vi "PWM.vi"(8 "Detener el PWM":bool, 9 "milliseconds to wait":u32, 10 "Ciclo de Trabajo":dbl(knob) scale=0.0..100.0, 11 "Frecuencia":dbl(knob) scale=0.0..100.0) -> (3 "Señal PWM":dbl(graph))   [LabVIEW 2018]
panel:
  # "Señal PWM"
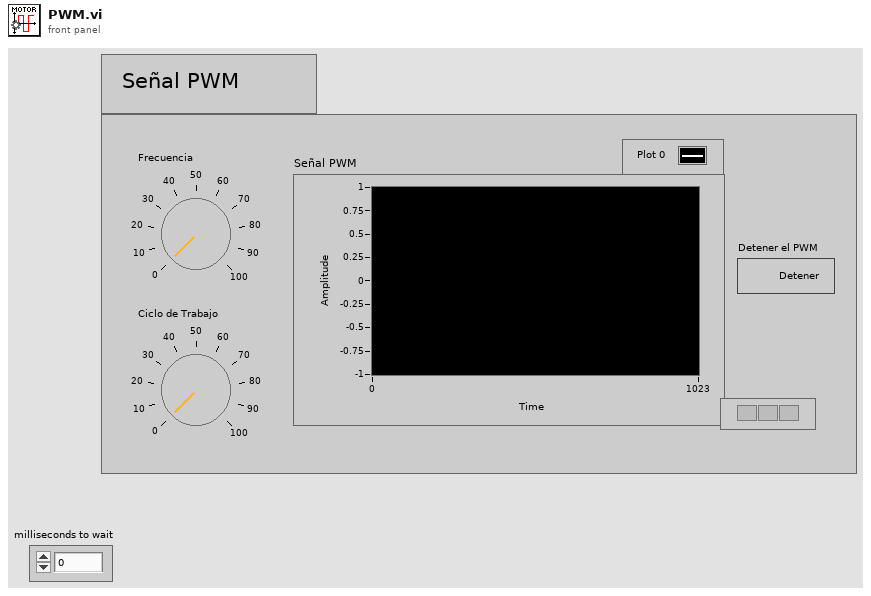
[diagram p1: front panel]
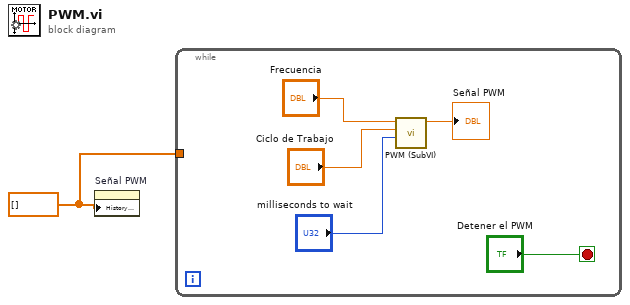
[diagram p0: block diagram]
diagram:
  w1 = dbl[] [] ("History Data")
  n1 = property on="Señal PWM" class="WFChart (strict)"("History Data"=w1) -> ()  [unwired: 2 in, 2 out]
  n2 = while {
    tunnel: w1 -> [_]
    stop <- "Detener el PWM" stop-if-true
    n3 = call "PWM (SubVI).vi"("milliseconds to wait"="milliseconds to wait", "Ciclo de Trabajo"="Ciclo de Trabajo", "Frecuencia"="Frecuencia") -> ("Señal PWM"=→"Señal PWM":dbl)  [unwired: 8 in]
  }
